vi "SP Read Parameters for Initialization.vi"(6 "Step Number":i32=1, 7 "S Parameter Test Parameters":T9={"Stimulus"={"Use Instrument Settings"=FALSE, "Blank Frequencies"=FALSE, "Sweep Type"=enum."Linear", "Sweep"={"Fstart"=500.0, "Fstop"=1500.0, "Units"=enum."MHz", "Points"=2}, "Power (dBm)"=999.0, "IFBW (Hz)"=-1.0, "Sweep Time (s)"=-1.0, "Calibration"={"State"=FALSE, "String"=""}}, "Measurement"={"Auto Select"=TRUE, "Data Source"=enum."VNA", "Ports"=2, "Parameters"=[]}, "De-Embed"={"De-Embed"=FALSE, "Adapters"=[]}, "Display"={"Lock Control"=FALSE, "Retain Settings"=TRUE, "Formatted Data"=FALSE, "Plot Orientation"=enum."Single", "Plot Controls"=[{"Trace Orientation"=enum."Overlay", "Frequency"={"Change Frequency"=FALSE, "Start"=500.0, "Stop"=1500.0, "Units"=enum."MHz"}, "Markers"=[], "Traces"=[]}, {"Trace Orientation"=enum."Overlay", "Frequency"={"Change Frequency"=FALSE, "Start"=500.0, "Stop"=1500.0, "Units"=enum."MHz"}, "Markers"=[], "Traces"=[]}, {"Trace Orientation"=enum."Overlay", "Frequency"={"Change Frequency"=FALSE, "Start"=500.0, "Stop"=1500.0, "Units"=enum."MHz"}, "Markers"=[], "Traces"=[]}, {"Trace Orientation"=enum."Overlay", "Frequency"={"Change Frequency"=FALSE, "Start"=500.0, "Stop"=1500.0, "Units"=enum."MHz"}, "Markers"=[], "Traces"=[]}]}, "Limits"=[], "Filter Limits"=[]} {"Filter Limits"."Parameter"."Stimulus Port" min=1 step=1; "Filter Limits"."Parameter"."Response Port" min=1 step=1; "Filter Limits"."Passband"."Bandwidth Attn" format="%.3g"; "Filter Limits"."Passband"."Stop/Span" format="%.3g"; "Filter Limits"."Passband"."Start/Center" format="%.3g"; "Measurement"."Parameters"."Channel" min=0 max=32 step=1; "Measurement"."Parameters"."Parameter"."Stimulus Port" min=1 step=1; "Measurement"."Parameters"."Parameter"."Response Port" min=1 step=1; "Limits"."Parameter"."Stimulus Port" min=1 step=1; "Limits"."Parameter"."Response Port" min=1 step=1; "Stimulus"."Sweep Time (s)" format="%.3g"; "Display"."Plot Controls"."Traces"."Reference" format="%#.2g"; "Display"."Plot Controls"."Traces"."Display Data" items=["Data", "Memory", "Data/Memory"]; "Display"."Plot Controls"."Traces"."Format" items=["Log Mag", "Phase", "Expanded Phase", "Delay", "Smith", "Polar", "Lin Mag", "SWR", "Loss", "Real", "Imaginary"]; "Display"."Plot Controls"."Traces"."Scale" min=0.001 step=1.0 format="%#.2g"; "Display"."Plot Controls"."Traces"."Position" min=0.0 max=10.0; "Display"."Plot Controls"."Frequency"."Stop" format="%.3g"; "Display"."Plot Controls"."Frequency"."Start" format="%.3g"}, 8 "error in (no error)":errorcluster, 9 "SNA? (F)":bool, 10 "Seq Count":i32, 11 "Channel Control Refs":refnum<vi>[](array[refnum])) -> (0 "error out":errorcluster, 2 "De-Embed Data":bool, 3 "Display":T1={"Lock Control"=FALSE, "Retain Settings"=TRUE, "Formatted Data"=FALSE, "Plot Orientation"=enum."Single", "Plot Controls"=[{"Trace Orientation"=enum."Overlay", "Frequency"={"Change Frequency"=FALSE, "Start"=500.0, "Stop"=1500.0, "Units"=enum."MHz"}, "Markers"=[], "Traces"=[]}, {"Trace Orientation"=enum."Overlay", "Frequency"={"Change Frequency"=FALSE, "Start"=500.0, "Stop"=1500.0, "Units"=enum."MHz"}, "Markers"=[], "Traces"=[]}, {"Trace Orientation"=enum."Overlay", "Frequency"={"Change Frequency"=FALSE, "Start"=500.0, "Stop"=1500.0, "Units"=enum."MHz"}, "Markers"=[], "Traces"=[]}, {"Trace Orientation"=enum."Overlay", "Frequency"={"Change Frequency"=FALSE, "Start"=500.0, "Stop"=1500.0, "Units"=enum."MHz"}, "Markers"=[], "Traces"=[]}]} {"Plot Controls"."Traces"."Reference" format="%#.2g"; "Plot Controls"."Traces"."Display Data" items=["Data", "Memory", "Data/Memory"]; "Plot Controls"."Traces"."Format" items=["Log Mag", "Phase", "Expanded Phase", "Delay", "Smith", "Polar", "Lin Mag", "SWR", "Loss", "Real", "Imaginary"]; "Plot Controls"."Traces"."Scale" min=0.001 step=1.0 format="%#.2g"; "Plot Controls"."Traces"."Position" min=0.0 max=10.0; "Plot Controls"."Frequency"."Stop" format="%.3g"; "Plot Controls"."Frequency"."Start" format="%.3g"})   [LabVIEW 2011]
uses:
  TypeDefs/SP Test Parameters.ctl
  TypeDefs/SP Stimulus Parameters.ctl
  TypeDefs/SP Frequency Units.ctl
  TypeDefs/SP Calibration State.ctl
  TypeDefs/SP Measurement.ctl
  TypeDefs/SP Parameters.ctl
  TypeDefs/SP Parameter.ctl
  TypeDefs/SP De-Embed.ctl
  TypeDefs/SP Adapter.ctl
  TypeDefs/SP Data.ctl
  TypeDefs/SP Display Parameters.ctl
  TypeDefs/SP Display Plot Controls Cluster.ctl
  TypeDefs/SP Marker Cluster.ctl
  TypeDefs/SP Marker Type.ctl
  TypeDefs/SP Display Trace Controls.ctl
  TypeDefs/SP Display Format.ctl
  TypeDefs/SP Display Data.ctl
  TypeDefs/SP Limit.ctl
  TypeDefs/SP Format.ctl
  TypeDefs/SP Limit Type.ctl
  TypeDefs/SP Limit Point.ctl
  Test Referential Limit.ctl
  TypeDefs/SP Filter.ctl
  TypeDefs/SP Filter Type.ctl
  TypeDefs/SP Filter Passband.ctl
  TypeDefs/SP Frequency Format.ctl
  TypeDefs/SP Filter Ripple.ctl
  TypeDefs/SP Attenuation Point.ctl
  TypeDefs/SP Attenuation Type.ctl
  TypeDefs/SP Skirt Rejection Point.ctl
  TypeDefs/SP Relative Loss.ctl
panel:
  # "Div"
  # "Div"
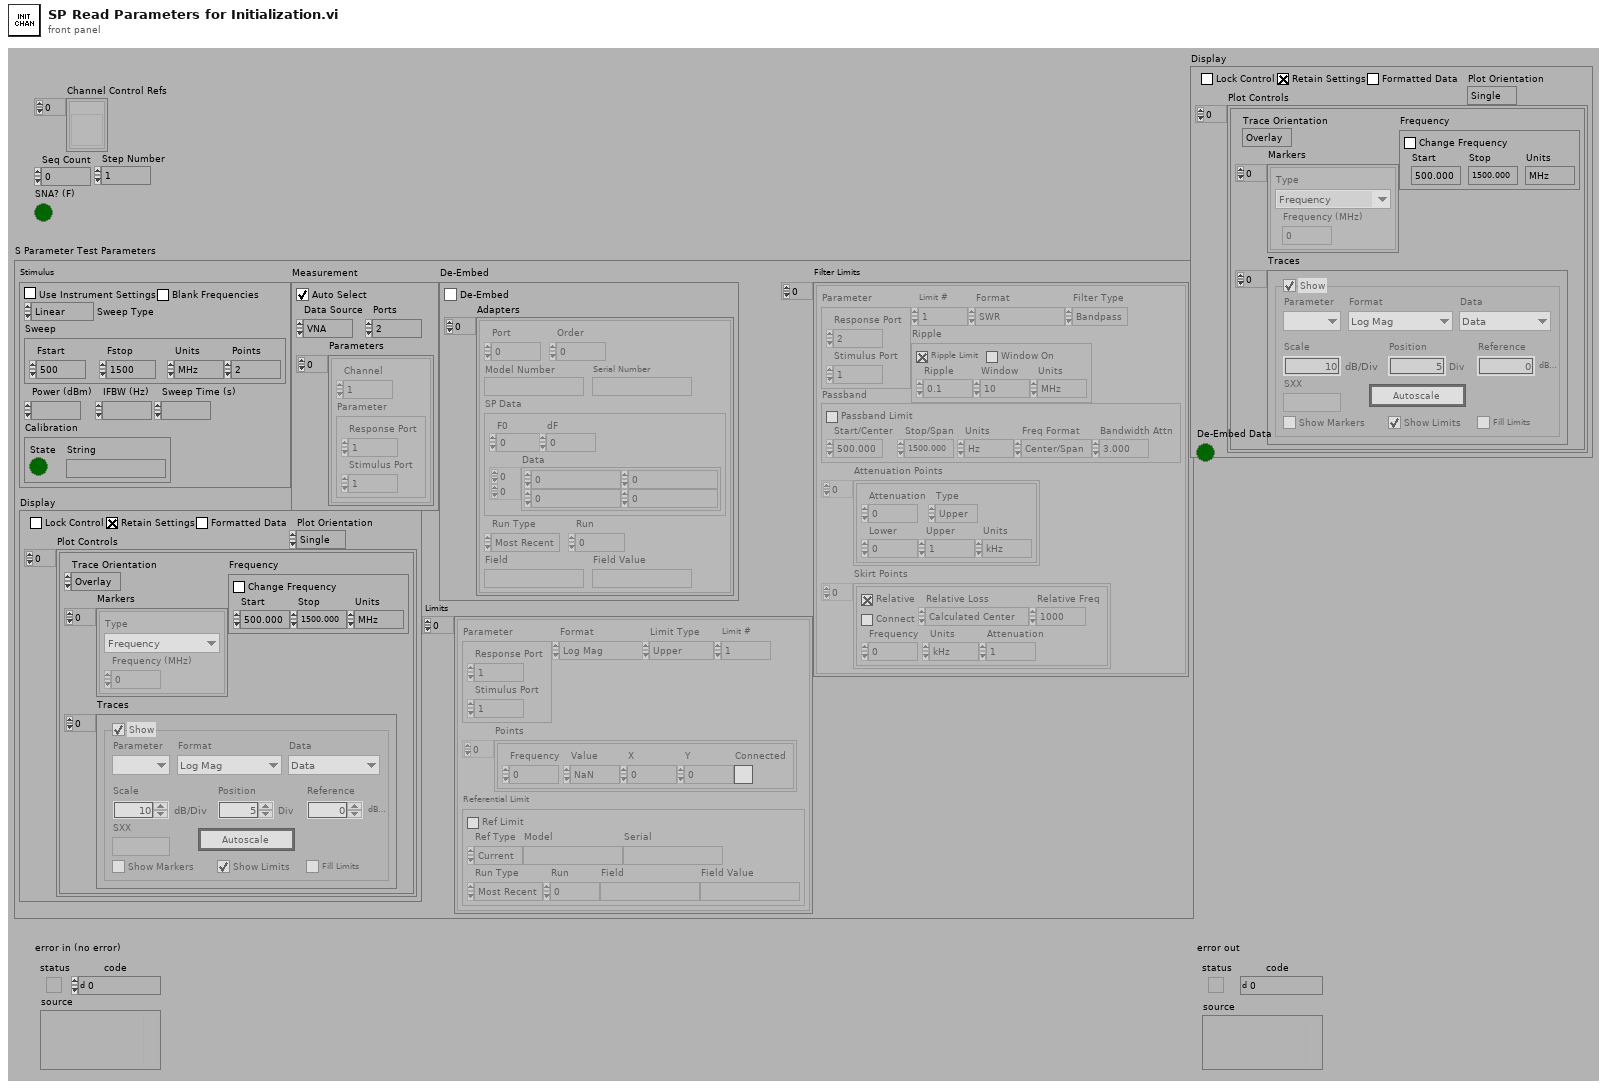
[diagram p1: front panel]
types:
  T1 = typedef "SP Display Parameters.ctl" = cluster{"Lock Control":bool, "Retain Settings":bool, "Formatted Data":bool, "Plot Orientation":enum32{"Single", "Dual", "Quad"}, "Plot Controls":T2[]}
  T2 = typedef "SP Display Plot Controls Cluster.ctl" = cluster{"Trace Orientation":enum32{"Overlay", "Split"}, "Frequency":cluster{"Change Frequency":bool, "Start":dbl, "Stop":dbl, "Units":T3}, "Markers":T4[], "Traces":T6[]}
  T3 = typedef "SP Frequency Units.ctl" = enum16{"Hz", "kHz", "MHz", "GHz", "Points"}
  T4 = typedef "SP Marker Cluster.ctl" = cluster{"Type":T5, "Frequency (MHz)":dbl}
  T5 = typedef "SP Marker Type.ctl" = enum16{"Frequency", "Trace Maximum", "Trace Minimum", "Limit Maximum", "Limit Minimum"}
  T6 = typedef "SP Display Trace Controls.ctl" = cluster{"Trace On":bool, "Measure":i32, "Format":T7, "Autoscale":bool, "Reference":dbl, "\nRefUnit":string, "Position":dbl, "Scale":dbl, "ScaleUnit":string, "LimitOn":bool, "LimitFill":bool, "Display Data":T8, "Show Markers":bool, "SXX":string}
  T7 = typedef "SP Display Format.ctl" = i32
  T8 = typedef "SP Display Data.ctl" = u16
  T9 = typedef "SP Test Parameters.ctl" = cluster{"Stimulus":T10, "Measurement":T12, "De-Embed":T15, "Display":T1, "Limits":T18[], "Filter Limits":T23[]}
  T10 = typedef "SP Stimulus Parameters.ctl" = cluster{"Use Instrument Settings":bool, "Blank Frequencies":bool, "Sweep Type":enum32{"Linear", "Logarithmic", "List", "Power", "CW"}, "Sweep":cluster{"Fstart":dbl, "Fstop":dbl, "Units":T3, "Points":i32}, "Power (dBm)":dbl, "IFBW (Hz)":dbl, "Sweep Time (s)":dbl, "Calibration":T11}
  T11 = typedef "SP Calibration State.ctl" = cluster{"State":bool, "String":string}
  T12 = typedef "SP Measurement.ctl" = cluster{"Auto Select":bool, "Data Source":enum16{"VNA", "Data File"}, "Ports":i8, "Parameters":T13[]}
  T13 = typedef "SP Parameters.ctl" = cluster{"Channel":i8, "Parameter":T14}
  T14 = typedef "SP Parameter.ctl" = cluster{"Stimulus Port":i8, "Response Port":i8}
  T15 = typedef "SP De-Embed.ctl" = cluster{"De-Embed":bool, "Adapters":T16[]}
  T16 = typedef "SP Adapter.ctl" = cluster{"Port":i8, "Order":i8, "Model Number":string, "Serial Number":string, "SP Data":T17, "Run Type":enum16{"Most Recent", "Run #", "Match Field"}, "Run":i32, "Field":string, "Field Value":string}
  T17 = typedef "SP Data.ctl" = cluster{"F0":dbl, "dF":dbl, "Data":cdb[][]}
  T18 = typedef "SP Limit.ctl" = cluster{"Parameter":T14, "Format":T19, "Limit Type":T20, "Points":T21[], "Referential Limit":T22, "Limit #":i8}
  T19 = typedef "SP Format.ctl" = enum16{"Log Mag", "Lin Mag", "SWR", "Phase", "Expanded Phase", "Delay", "Insertion Loss", "Isolation", "Return Loss"}
  T20 = typedef "SP Limit Type.ctl" = enum16{"Upper", "Lower", "Delta", "Filter", "Referential"}
  T21 = typedef "SP Limit Point.ctl" = cluster{"Frequency":dbl, "Value":dbl, "X":dbl, "Y":dbl, "Connected":bool}
  T22 = typedef "Test Referential Limit.ctl" = cluster{"Ref Limit":bool, "Ref Type":enum16{"Current", "Specify"}, "Model":string, "Serial":string, "Run Type":enum16{"Most Recent", "Run #", "Match Field"}, "Run":i32, "Field":string, "Field Value":string}
  T23 = typedef "SP Filter.ctl" = cluster{"Limit #":i8, "Parameter":T14, "Format":T19, "Filter Type":T24, "Passband":T25, "Ripple":T27, "Attenuation Points":T28[], "Skirt Points":T30[]}
  T24 = typedef "SP Filter Type.ctl" = enum16{"Lowpass", "Highpass", "Bandpass", "Bandstop"}
  T25 = typedef "SP Filter Passband.ctl" = cluster{"Start/Center":dbl, "Stop/Span":dbl, "Units":T3, "Freq Format":T26, "Bandwidth Attn":dbl, "Passband Limit":bool}
  T26 = typedef "SP Frequency Format.ctl" = enum16{"Start/Stop", "Center/Span"}
  T27 = typedef "SP Filter Ripple.ctl" = cluster{"Ripple Limit":bool, "Window On":bool, "Ripple":dbl, "Window":dbl, "Units":T3}
  T28 = typedef "SP Attenuation Point.ctl" = cluster{"Attenuation":dbl, "Type":T29, "Lower":dbl, "Upper":dbl, "Units":T3}
  T29 = typedef "SP Attenuation Type.ctl" = enum16{"Center", "Lower", "Upper"}
  T30 = typedef "SP Skirt Rejection Point.ctl" = cluster{"Relative":bool, "Connect":bool, "Frequency":dbl, "Units":T3, "Attenuation":dbl, "Relative Loss":T31, "Relative Freq":dbl}
  T31 = typedef "SP Relative Loss.ctl" = enum16{"Calculated Center", "Passband Minimum", "Passband Maximum", "Passband Average", "Frequency"}
  T32 = cluster{"Fstart":dbl, "Fstop":dbl, "Units":T3, "Points":i32}
  T33 = enum8{"Enabled", "Disabled", "Disabled and Grayed Out"}
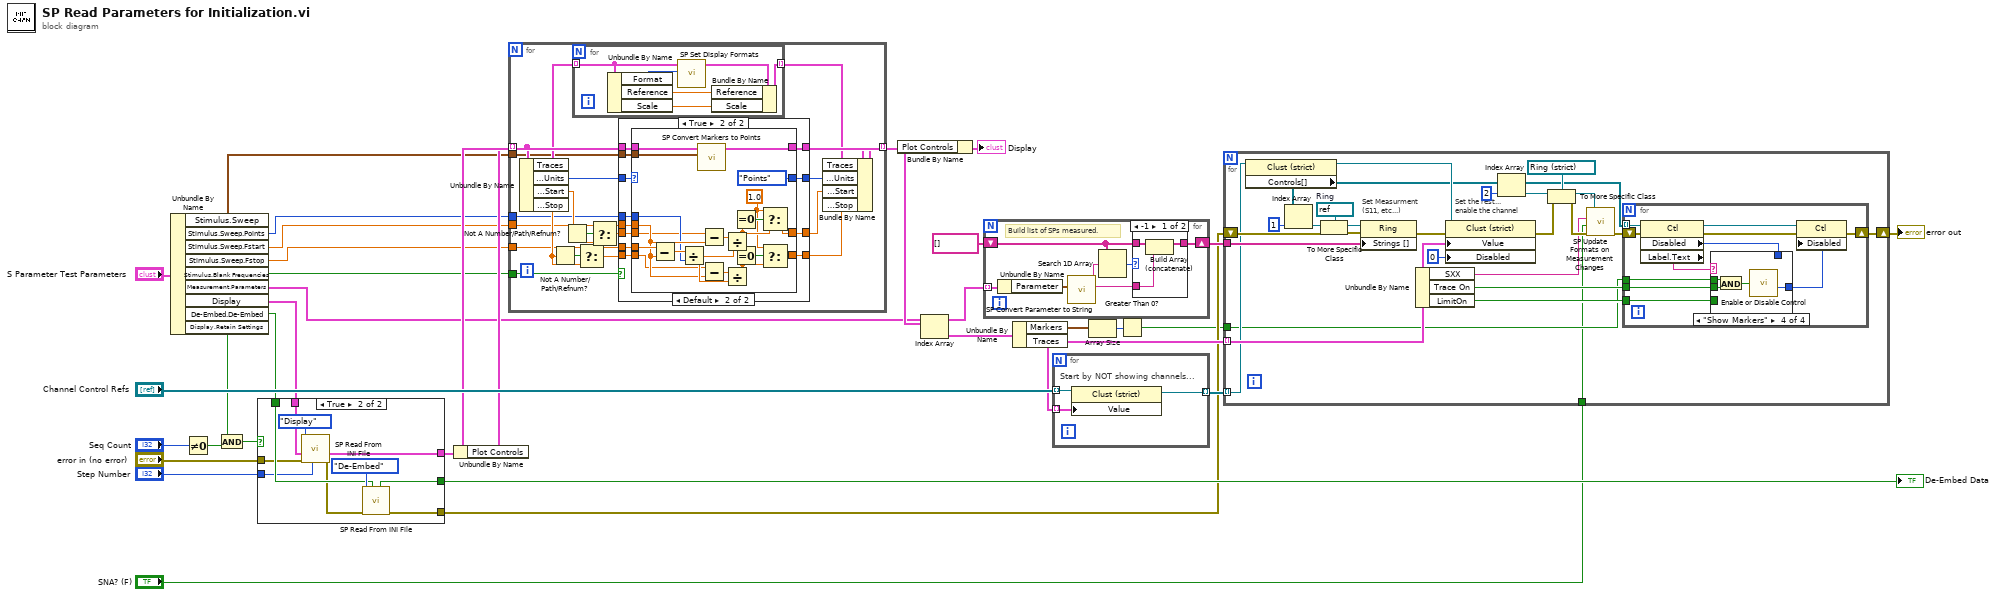
[diagram p0: block diagram]
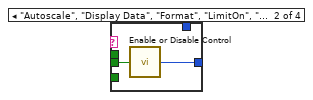
[diagram p7: hidden frame]
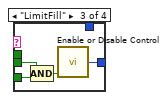
[diagram p8: hidden frame]
diagram:
  n1 = Unbundle By Name("S Parameter Test Parameters") -> ("Stimulus.Sweep"=w8:T32, "Stimulus.Sweep.Points"=w12:i32, "Stimulus.Sweep.Fstart"=w7:dbl, "Stimulus.Sweep.Fstop"=w6:dbl, "Stimulus.Blank Frequencies"=w13:bool, "Measurement.Parameters"=w5:T13[], "Display"=w4:T1, "De-Embed.De-Embed"=w3:bool, "Display.Retain Settings"=w27:bool)
  n2 = Not Equal To 0?(x="Seq Count") -> (x != 0?=w28:bool)
  n3 = And(x=w27, y=w28) -> (x .and. y?=w26:bool)
  n4 = case shown="True" w26 {
    tunnel: [w35 w45] -> w24
    tunnel: w4 -> [w35 w44]
    tunnel: w3 -> [w34 w41]
    tunnel: [w34 w40] -> w19
    tunnel: "error in (no error)" -> [w33 w39]
    tunnel: [w33 w37] -> w16
    tunnel: "Step Number" -> [_ w36]
    frame False {
    }
    frame True {
      n5 = call "SP Read From INI File.vi"("Step Number"=w36, "error in (no error)"=w39, "Display In"=w44, "Data to Read"=enum16{"Calibration", "Display", "De-Embed"}."Display") -> ("error out"=w38:errorcluster, "Display Out"=w45:T1)  [unwired: 2 in, 4 out]
      n6 = call "SP Read From INI File.vi"("De-Embed Data In"=w41, "error in (no error)"=w38, "Data to Read"=enum16{"Calibration", "Display", "De-Embed"}."De-Embed") -> ("error out"=w37:errorcluster, "De-Embed Data Out"=w40:bool)  [unwired: 3 in, 4 out]
    }
  }
  "De-Embed Data" <- w19
  n7 = Unbundle By Name(w24) -> ("Plot Controls"=w15:T2[])
  n8 = for {
    tunnel: w15 -> [w49] mode=indexing
    tunnel: [w65] -> w14 mode=indexing
    tunnel: w7 -> [w52]
    tunnel: w6 -> [w51]
    tunnel: w13 -> [w58]
    tunnel: w12 -> [w50]
    tunnel: w8 -> [w47]
    n9 = Unbundle By Name(w49) -> ("Traces"=w60:T6[], "Frequency.Units"=w46:T3, "Frequency.Start"=w63:dbl, "Frequency.Stop"=w61:dbl)
    n10 = Not A Number/Path/Refnum?(number/path/refnum=w61) -> (NaN/Path/Refnum?=w62:bool)
    n11 = Not A Number/Path/Refnum?(number/path/refnum=w63) -> (NaN/Path/Refnum?=w64:bool)
    n12 = for {
      tunnel: w60 -> [w111] mode=indexing
      tunnel: [w109] -> w59 mode=indexing
      n13 = Unbundle By Name(w111) -> ("Format"=w106:T7, "Reference"=w108:dbl, "Scale"=w107:dbl)
      n14 = call "SP Set Display Formats.vi"("Format"=w106, "CH Controls"=w111) -> ("new CH Controls"=w110:T6)  [unwired: 1 in, 8 out]
      n15 = Bundle By Name(cluster=w110, "Reference"=w108, "Scale"=w107) -> (w109:T6)
    }
    n16 = Select(t=w51, s=w62, f=w61) -> (s? t:f=w57:dbl)
    n17 = Select(t=w52, s=w64, f=w63) -> (s? t:f=w55:dbl)
    n18 = case shown="True" w58 {
      tunnel: w55 -> [w68 w72]
      tunnel: w57 -> [w69 w71]
      tunnel: [w69 w78] -> w56
      tunnel: [w68 w79] -> w54
      tunnel: w46 -> [w67 w70]
      tunnel: [w67 w81] -> w53
      tunnel: w52 -> [_ w77]
      tunnel: w51 -> [_ w80]
      tunnel: w50 -> [_ w76]
      tunnel: w49 -> [w66 w75]
      tunnel: [w66 w74] -> w48
      tunnel: w47 -> [_ w73]
      frame False {
      }
      frame True {
        n19 = case shown="Default" w70 {
          selector: w70 -> [w83 _]
          tunnel: [w83 SP_Frequency_Units."Points" ("Units")] -> w81
          tunnel: w80 -> [_ w104]
          tunnel: [w85 w97] -> w79
          tunnel: [w84 w96] -> w78
          tunnel: w77 -> [_ w93]
          tunnel: w76 -> [_ w91]
          tunnel: w75 -> [w82 w90]
          tunnel: [w82 w89] -> w74
          tunnel: w73 -> [_ w88]
          tunnel: w72 -> [w85 w87]
          tunnel: w71 -> [w84 w86]
          frame "Points" {
          }
          frame Default {
            w94 = 1.0 ("t")
            n20 = Subtract(x=w104, y=w93) -> (x-y=w92:dbl)
            n21 = Divide(x=w92, y=w91) -> (x/y=w101:dbl)
            n22 = call "SP Convert Markers to Points.vi"("Sweep"=w88, "Plot Control In"=w90) -> ("Plot Control Out"=w89:T2)  [unwired: 9 out]
            n23 = Subtract(x=w87, y=w93) -> (x-y=w103:dbl)
            n24 = Subtract(x=w86, y=w93) -> (x-y=w102:dbl)
            n25 = Divide(x=w103, y=w101) -> (x/y=w98:dbl)
            n26 = Divide(x=w102, y=w101) -> (x/y=w95:dbl)
            n27 = Equal To 0?(x=w98) -> (x = 0?=w100:bool)
            n28 = Equal To 0?(x=w95) -> (x = 0?=w99:bool)
            n29 = Select(t=w94, s=w100, f=w98) -> (s? t:f=w97:dbl)
            n30 = Select(t=w94, s=w99, f=w95) -> (s? t:f=w96:dbl)
          }
        }
      }
    }
    n31 = Bundle By Name(cluster=w48, "Traces"=w59, "Frequency.Units"=w53, "Frequency.Start"=w54, "Frequency.Stop"=w56) -> (w65:T2)
  }
  n32 = Bundle By Name(cluster=w24, "Plot Controls"=w14) -> (→"Display":T1)
  n33 = Index Array(array=w14) -> (element=w25:T2)  [unwired: 1 in]
  n34 = for {
    tunnel: w5 -> [w117] mode=indexing
    shift-right: [w112] -> w21
    shift-left: string[] [] -> [w114]
    # "Build list of SPs measured."
    n35 = Unbundle By Name(w117) -> ("Parameter"=w116:T14)
    n36 = call "SP Convert Parameter to String.vi"("Parameter"=w116) -> ("Parameter String"=w113:string)  [unwired: 10 out]
    n37 = Search 1D Array(1D array=w114, element=w113) -> (index of element=w115:i32)  [unwired: 1 out]
    n38 = case shown="-1" w115 {
      tunnel: w114 -> [w120 w121]
      tunnel: w113 -> [w119 _]
      tunnel: [w118 w121] -> w112
      frame -1 {
        n39 = Build Array (concatenate)(w120, w119) -> (w118:string[])
      }
      frame Default {
      }
    }
  }
  n40 = Unbundle By Name(w25) -> ("Markers"=w11:T4[], "Traces"=w20:T6[])
  n41 = for {
    tunnel: "Channel Control Refs" -> [w124] mode=indexing
    tunnel: [w123] -> w31 mode=indexing
    tunnel: w20 -> [w122] mode=indexing
    # "Start by NOT showing channels..."
    n42 = property class="Clust (strict)"(reference=w124, "Value"=w122) -> (reference out=w123:refnum<vi>)  [unwired: 1 in, 1 out]
  }
  n43 = Array Size(array=w11) -> (size(s)=w10:i32)
  n44 = Greater Than 0?(x=w10) -> (x > 0?=w9:bool)
  n45 = for {
    tunnel: w31 -> [w131] mode=indexing
    tunnel: w20 -> [w132] mode=indexing
    tunnel: w21 -> [w142]
    shift-right: [w128] -> w17
    shift-left: w16 -> [w141]
    tunnel: w9 -> [w130]
    tunnel: "SNA? (F)" -> [w125]
    w147 = refnum<vi> refnum  # Ring
    # "Set the rest...\nenable the channel"
    # "Set Measurment\n(S11, etc...)"
    n46 = property class="Clust (strict)"(reference=w131) -> (reference out=w148:refnum<vi>, "Controls[]"=w127:refnum<vi>[])  [unwired: 1 in, 1 out]
    n47 = Index Array(array=w127, index=1) -> (element=w146:refnum<vi>)
    n48 = To More Specific Class(target class=w147, reference=w146, error in=w141) -> (specific class reference=w145:refnum<vi>, error out=w140:errorcluster)
    n49 = property class="Ring"(reference=w145, error in=w140, "Strings []"=w142) -> (error out=w135:errorcluster)  [unwired: 1 out]
    n50 = Unbundle By Name(w132) -> ("SXX"=w126:string, "Trace On"=w133:bool, "LimitOn"=w134:bool)
    n51 = property class="Clust (strict)"(reference=w148, error in=w135, "Value"=w132, "Disabled"=u8 0) -> (error out=w137:errorcluster)  [unwired: 1 out]
    n52 = Index Array(array=w127, index=2) -> (element=w143:refnum<vi>)
    n53 = To More Specific Class(target class=refnum<vi> refnum ("Format"), reference=w143, error in=w137) -> (specific class reference=w138:refnum<vi>, error out=w136:errorcluster)
    n54 = call "SP Update Formats on Measurement Changes.vi"("error in (no error)"=w136, "SNA? (F)"=w125, "Parameter String"=w126, "Format"=w138) -> ("error out"=w129:errorcluster)  [unwired: 3 out]
    n55 = for {
      shift-right: [w157] -> w128
      shift-left: w129 -> [w160]
      tunnel: w127 -> [w161] mode=indexing
      tunnel: w133 -> [w159]
      tunnel: w134 -> [w158]
      tunnel: w130 -> [w151]
      n56 = property class="Ctl"(reference=w161, error in=w160) -> (reference out=w156:refnum<vi>, error out=w154:errorcluster, "Disabled"=w152:u8, "Label.Text"=w153:string)
      n57 = case shown="\"Show Markers\"" w153 {
        tunnel: w159 -> [_ w164 w168 w171]
        tunnel: w158 -> [_ _ w167 _]
        tunnel: [w162 w163 w165 w172] -> w155
        tunnel: w152 -> [w162 _ _ _]
        tunnel: w151 -> [_ _ _ w169]
        frame Default {
        }
        frame "Autoscale", "Display Data", "Format", "LimitOn", "Measure", "Position", "Reference", "Scale" {
          n58 = call "Enable or Disable Control.vi"("Enable? (T)"=w164) -> ("Enable\\Disable"=w163:T33)
        }
        frame "LimitFill" {
          n59 = Compound Arithmetic op=AND(w168, w167) -> (w166:bool)
          n60 = call "Enable or Disable Control.vi"("Enable? (T)"=w166) -> ("Enable\\Disable"=w165:T33)
        }
        frame "Show Markers" {
          n61 = And(x=w169, y=w171) -> (x .and. y?=w170:bool)
          n62 = call "Enable or Disable Control.vi"("Enable? (T)"=w170) -> ("Enable\\Disable"=w172:T33)
        }
      }
      n63 = property class="Ctl"(reference=w156, error in=w154, "Disabled"=w155) -> (error out=w157:errorcluster)  [unwired: 1 out]
    }
  }
  "error out" <- w17
